vi "IMAQ-MWT DMD XY Calibration (HOST).vi"() -> ()   [LabVIEW 2015]
uses:
  Modules/Common/Controls (HOST)/Image Size.ctl
  Modules/Common/Controls (HOST)/REF.ctl
  Modules/Common/Controls (HOST)/Image Queue Bundle.ctl
  Modules/Common/Controls (HOST)/Data to Disk Bundle.ctl
  Modules/Common/Controls (HOST)/FPGA REF (MWT).ctl
  Modules/Common/Controls (HOST)/Experiment Mode.ctl
  Modules/Common/Controls (HOST)/Main States.ctl
  Modules/Common/Controls (HOST)/IMAQ Parameters.ctl
  Modules/Common/Controls (HOST)/File REF.ctl
  <vilib>/vision/Avi.llb/IMAQ AVI2 Refnum.ctl
  <vilib>/Utility/error.llb/Error Cluster From Error Code.vi
  <vilib>/rvi/errors/niLvFpgaAdjustHostInterfaceError.vi
  <vilib>/FPGAPlugInAG/Dynamic/niLvFpga_Close_Dynamic.vi
  <vilib>/Utility/file.llb/Write Delimited Spreadsheet (I64).vi
  <vilib>/rvi/interface/nirviReadWriteControl/nirviReadWriteControl.xnode
  <vilib>/rvi/interface/nirviCloseFPGA/nirviCloseFPGA.xnode
  NiFpgaLv.dll
  <vilib>/rvi/interface/Simulation/niFpgaSimulationCallBeginRW.vi
  <vilib>/Utility/config.llb/NI_LVConfig.lvlib
  <vilib>/vision/NI_Vision_Development_Module.lvlib
  <vilib>/Utility/config.llb/Write Key (U32).vi
panel:
  out "DMD (Center)":cluster{"X":i32, "Y":i32}={"X"=400, "Y"=300}
  out "Cam (Center)":cluster{"X":i32, "Y":i32}
  in  "DMD ( Top/Left)":cluster{"X":i32, "Y":i32}={"X"=295, "Y"=95}
  in  "DMD #":enum16{"DMD1", "DMD2"}(ring)
  in  "Tab Control":enum32{"Setup", "X Axis", "Y Axis"}(tab)
  in  "Image Size":T1={"Height"=3072, "Width"=3200}
  in  "Experiment Mode":T2
  in  "Pixel Intensity Range":cluster{"Low":u8, "High":u8}={"Low"=25, "High"=135}
  in  "Exp. Time (S)":dbl=120.0
  in  "Stop Button":bool
  in  "Go":bool
  in  "Subtract BG":bool=TRUE
  in  "Replay Interval (ms)":u32=1000
  in  "Swap Bytes":bool
  in  "BOX Height":i32=10
  in  "BOX Width":i32=10
  in  "DMD Height":i32=768
  in  "DMD Width":i32=1024
  out "Particle Reports (Pixels)":T3(array[cluster]) {"Orientation" format="%.2f"; "Dimensions"."Height" format="%.2f"; "Dimensions"."Width" format="%.2f"; "Center of Mass"."Y" format="%.2f"; "Center of Mass"."X" format="%.2f"; "Bounding Rect"."Bottom" format="%.2f"; "Bounding Rect"."Right" format="%.2f"; "Bounding Rect"."Top" format="%.2f"; "Bounding Rect"."Left" format="%.2f"; "Number of Holes" format="%.2f"; "Area" format="%.2f"}
  in  "Range":cluster{"Low":sgl, "High":sgl}={"Low"=150.0, "High"=255.0}
  in  "Selection Values":T5(array[cluster])=[{"Measurement Parameter"=18, "Range Lower Value"=50.0, "Range Upper Value"=1000.0, "Range"=FALSE, "Measurement Type"=FALSE}] {"Measurement Parameter" items=["Center of Mass X", "Center of Mass Y", "First Pixel X", "First Pixel Y", "Bounding Rect Left", "Bounding Rect Top", "Bounding Rect Right", "Bounding Rect Bottom", "Max Feret Diameter Start X", "Max Feret Diameter Start Y", "Max Feret Diameter End X", "Max Feret Diameter End Y", "Max Horiz. Segment Length Left", "Max Horiz. Segment Length Right", "Max Horiz. Segment Length Row", "-", "Bounding Rect Width", "Bounding Rect Height", "Bounding Rect Diagonal", "Perimeter", "Convex Hull Perimeter", "Holes' Perimeter", "Max Feret Diameter", "Equivalent Ellipse Major Axis", "Equivalent Ellipse Minor Axis", "Equivalent Ellipse Minor Axis (Feret)", "Equivalent Rect Long Side", "Equivalent Rect Short Side", "Equivalent Rect Diagonal", "Equivalent Rect Short Side (Feret)", "Average Horiz. Segment Length", "Average Vert. Segment Length", "Hydraulic Radius", "Waddel Disk Diameter", "-", "Area", "Holes' Area", "Particle & Holes' Area", "Convex Hull Area", "Image Area", "-", "Number of Holes", "Number of Horiz. Segments", "Number of Vert. Segments", "-", "Orientation", "Max Feret Diameter Orientation", "-", "% Area/Image Area", "% Area/(Particle & Holes' Area)", "Ratio of Equivalent Ellipse Axes", "Ratio of Equivalent Rect Sides", "-", "Elongation Factor", "Compactness Factor", "Heywood Circularity Factor", "Type Factor", "-", "Sum X", "Sum Y", "Sum XX", "Sum XY", "Sum YY", "Sum XXX", "Sum XXY", "Sum XYY", "Sum YYY", "-", "Moment of Inertia XX", "Moment of Inertia XY", "Moment of Inertia YY", "Moment of Inertia XXX", "Moment of Inertia XXY", "Moment of Inertia XYY", "Moment of Inertia YYY", "Norm. Moment of Inertia XX", "Norm. Moment of Inertia XY", "Norm. Moment of Inertia YY", "Norm. Moment of Inertia XXX", "Norm. Moment of Inertia XXY", "Norm. Moment of Inertia XYY", "Norm. Moment of Inertia YYY", "Hu Moment 1", "Hu Moment 2", "Hu Moment 3", "Hu Moment 4", "Hu Moment 5", "Hu Moment 6", "Hu Moment 7"]; "Range Lower Value" format="%.2f"; "Range Upper Value" format="%.2f"}
  out "Number of Particles":i32
  out "Frame #":u32
  out "Frame Rate":u32
  in  "Movie File Path":path=path "E:/Rawdata/72F11-Gal4xUAS-CsChrimson_20180513_192634.dbde"
  in  "DMD (X Axis)":i32[][](array[numeric])=[[300, 100], [900, 100], [900, 650], [300, 650]]
  in  "Camera (X Axis)":i32[][](array[numeric])
  in  "Save X Table":bool
  in  "Save GUI Parameters":bool
  in  "Gamma":dbl=0.2 format="%#_13g"
  in  "Min Contour Points":u16=127
  in  "N Spine Points":fxp<+,8,8>=41.0
  in  "BG SUB TH":i16=10
  in  "Save Y Table":bool
  in  "DMD (Y Axis)":i32[][](array[numeric])=[[500, 100], [500, 200], [500, 300], [500, 400], [500, 500], [500, 600], [500, 700], [500, 800]]
  in  "Camera (Y Axis)":i32[][](array[numeric])
  out "Exp. Status":string="Camera Connected"
  out "REF":T6
  out "Command Q":refnum<queue>
  out "Display":T9(plugin-control)
  out "Stopped?":bool
  # "DMD XY Calibration"
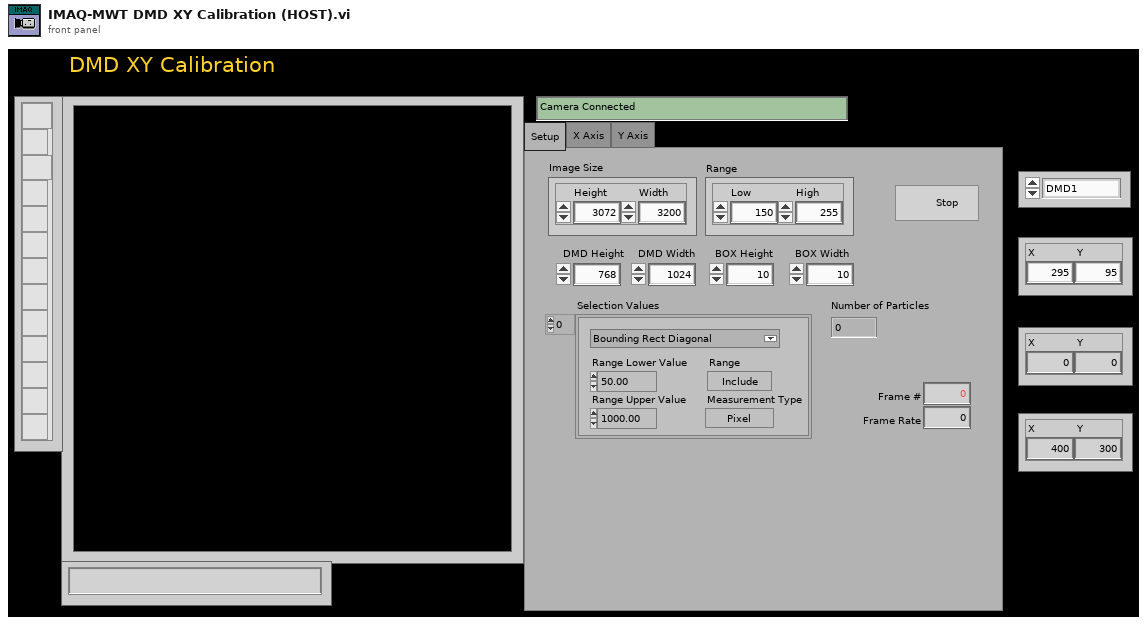
[diagram p1: front panel]
types:
  T1 = typedef "Image Size.ctl" = cluster{"Height":u16, "Width":u16}
  T2 = typedef "Experiment Mode.ctl" = enum16{"Live", "Replay"}
  T3 = cluster{"Area":dbl, "Number of Holes":dbl, "Bounding Rect":cluster{"Left":dbl, "Top":dbl, "Right":dbl, "Bottom":dbl}, "Center of Mass":cluster{"X":dbl, "Y":dbl}, "Orientation":dbl, "Dimensions":cluster{"Width":dbl, "Height":dbl}}[]
  T4 = typedef "Particle Parameters" = i32
  T5 = cluster{"Measurement Parameter":T4, "Range Lower Value":dbl, "Range Upper Value":dbl, "Range":bool, "Measurement Type":bool}[]
  T6 = typedef "REF.ctl" = cluster{"Queue REF":T7, "FPGA REF (MWT)":T8}
  T7 = typedef "Image Queue Bundle.ctl" = cluster{"Disk Image":refnum<queue>, "Image Blocks":refnum<queue>, "Display Image":refnum<queue>, "BG Image":refnum<queue>, "Tag Image":refnum<queue>}
  T8 = typedef "FPGA REF (MWT).ctl" = refnum<k20>
  T9 = typedef "IMAQ Image.ctl" = refnum<image>
  T10 = enum8{"Enabled", "Disabled", "Disabled and Grayed Out"}
  T11 = typedef "Main States.ctl" = enum16{"Open FPGA", "Initialize", "Preview", "Acquire Images", "STOP"}
  T12 = typedef "IMAQ Parameters.ctl" = cluster{"File REF":T13, "Frame Data":cluster{"Width":u32, "Height":u32, "Frames Per Second":u32, "Codec":string}, "File Type":string, "Experiment Mode":T2, "Movie File Path":path}
  T13 = typedef "File REF.ctl" = cluster{"AVI REF":T14, "DBDE REF":refnum<file>}
  T14 = typedef "IMAQ AVI2 Refnum.ctl" = refnum<k20>
  T15 = typedef "Data to Disk Bundle.ctl" = cluster{"Frame Number":u64, "Time Stamp (us)":u64, "Image Data":u64[], "Contour":u32[], "Raw Image REF":refnum<data-value>, "Block Image REF":refnum<data-value>, "Block Box":u64[], "SPINE":u32[], "HT Angle":u64[], "Block Position":u64[], "SPINE Count":u32[], "Contour Count":u32[], "SPINE DIR":u8[]}
  T16 = cluster{"Area":dbl, "Number of Holes":dbl, "Bounding Rect":cluster{"Left":dbl, "Top":dbl, "Right":dbl, "Bottom":dbl}, "Center of Mass":cluster{"X":dbl, "Y":dbl}, "Orientation":dbl, "Dimensions":cluster{"Width":dbl, "Height":dbl}}
  T17 = cluster{"Left":dbl, "Top":dbl, "Right":dbl, "Bottom":dbl}
  T18 = typedef "NI_LVConfig.lvlib/Config Data RefNum.ctl" = refnum<k1>
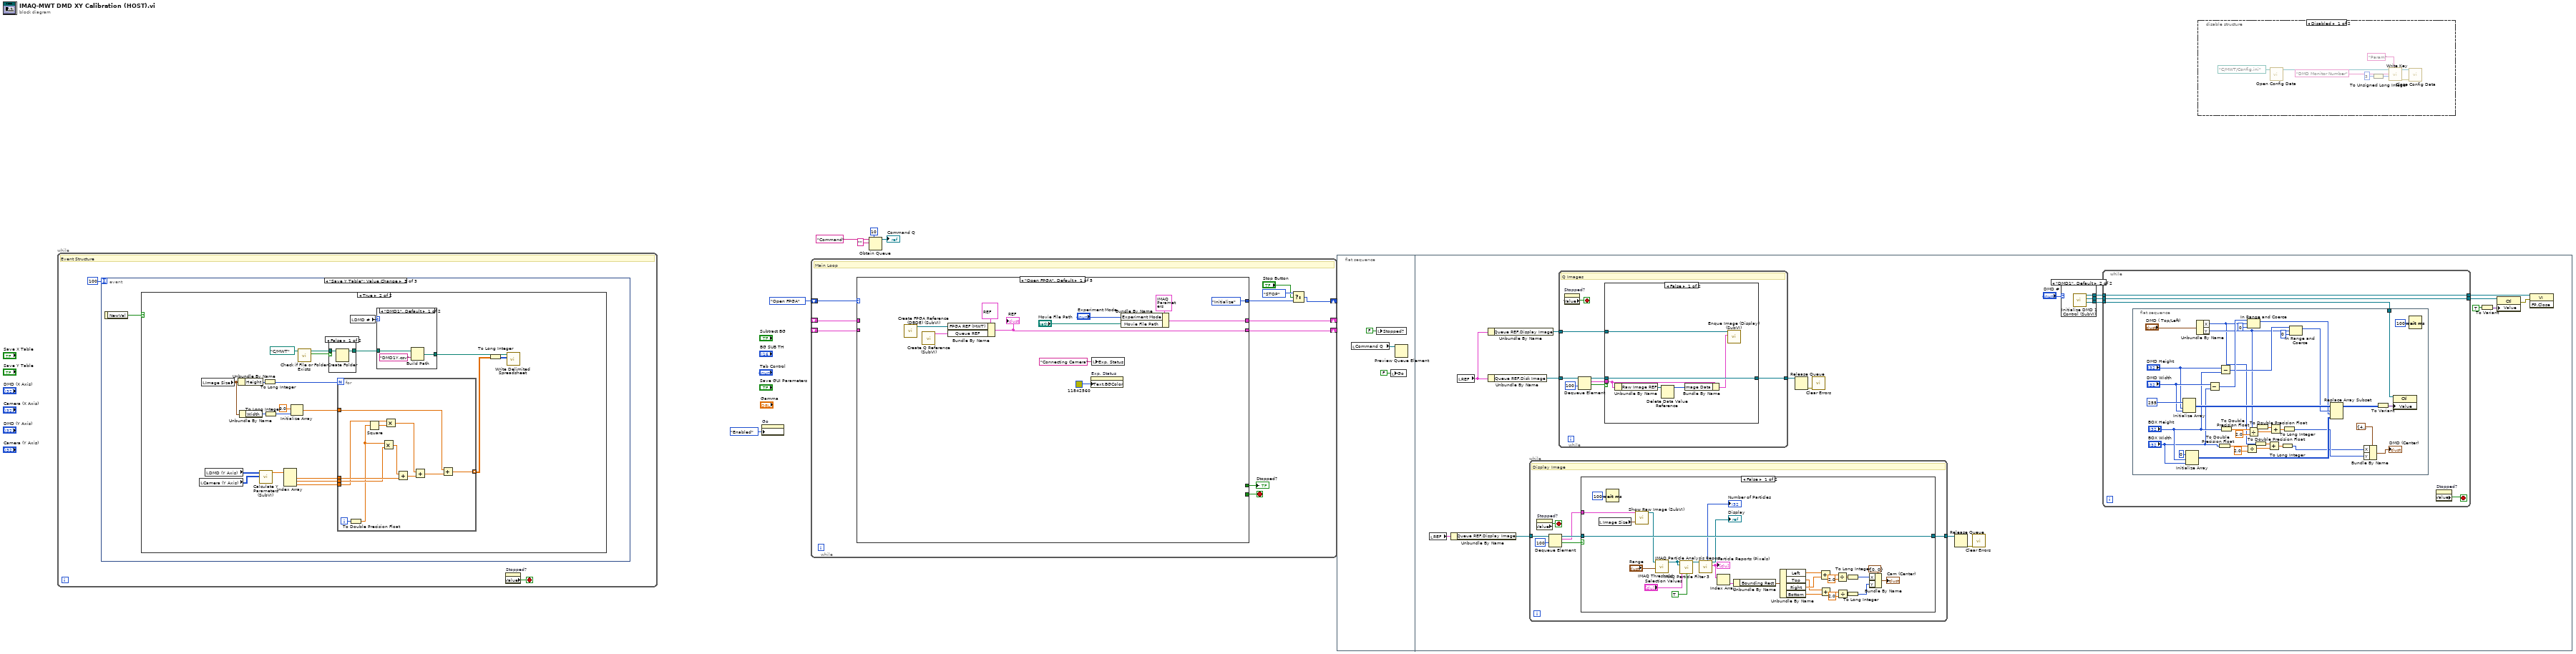
[diagram p0: block diagram]
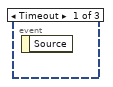
[diagram p2: hidden frame]
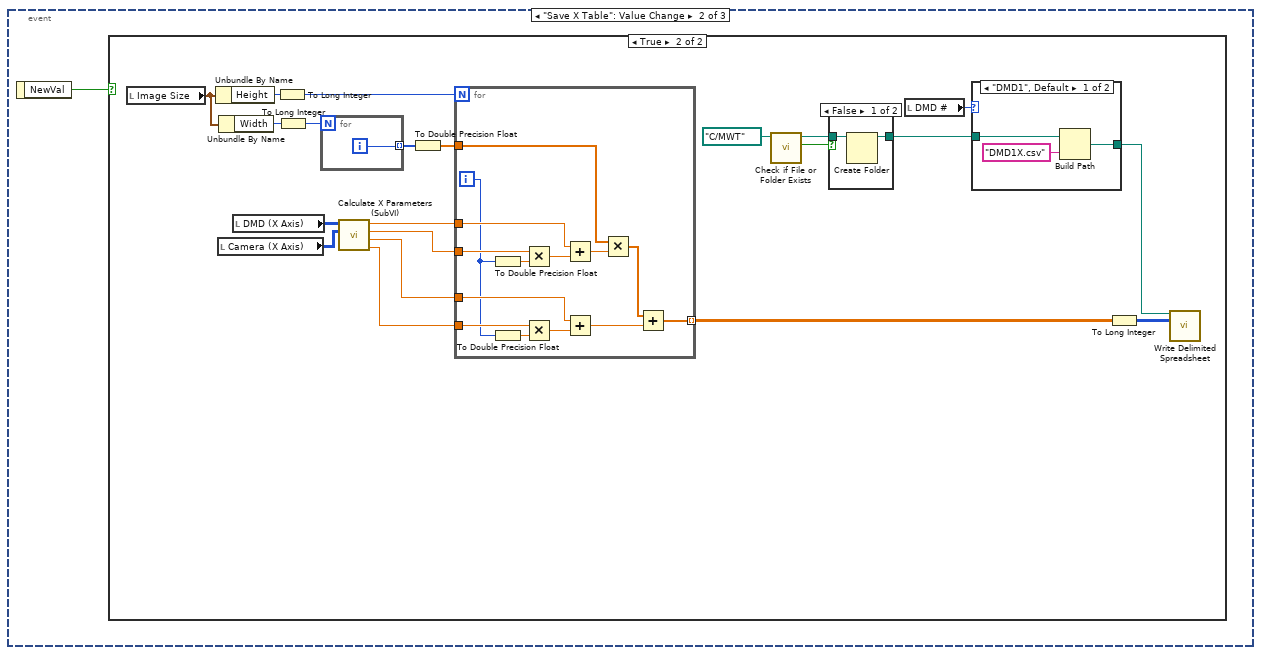
[diagram p3: hidden frame]
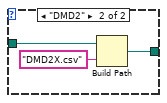
[diagram p6: hidden frame]
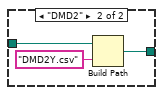
[diagram p9: hidden frame]
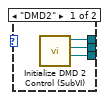
[diagram p11: hidden frame]
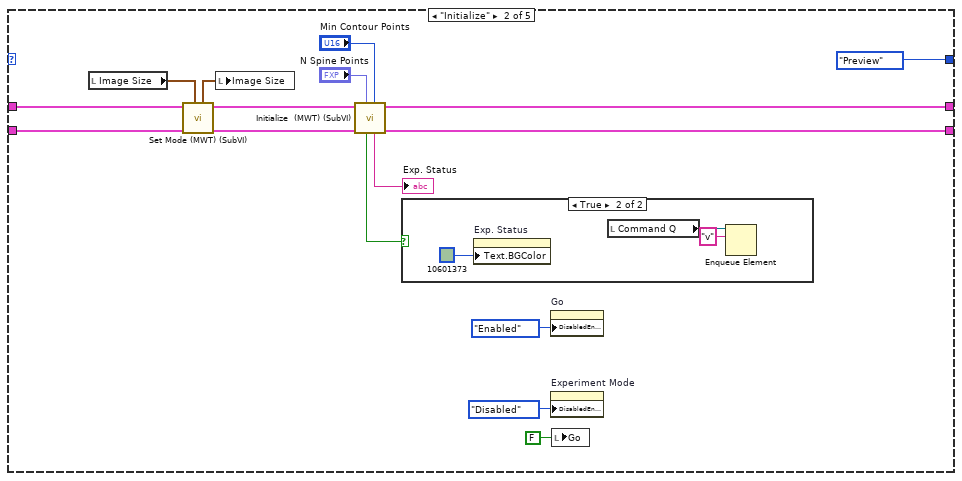
[diagram p14: hidden frame]
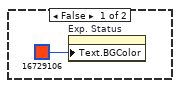
[diagram p15: hidden frame]
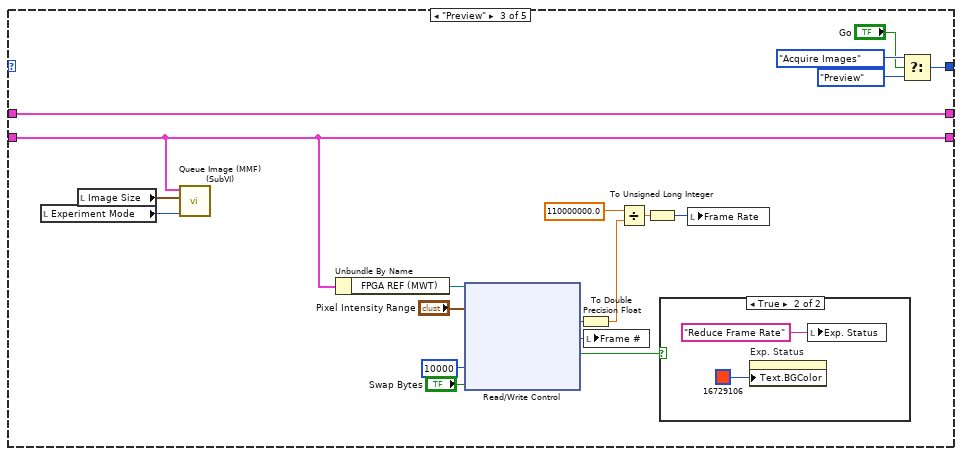
[diagram p16: hidden frame]
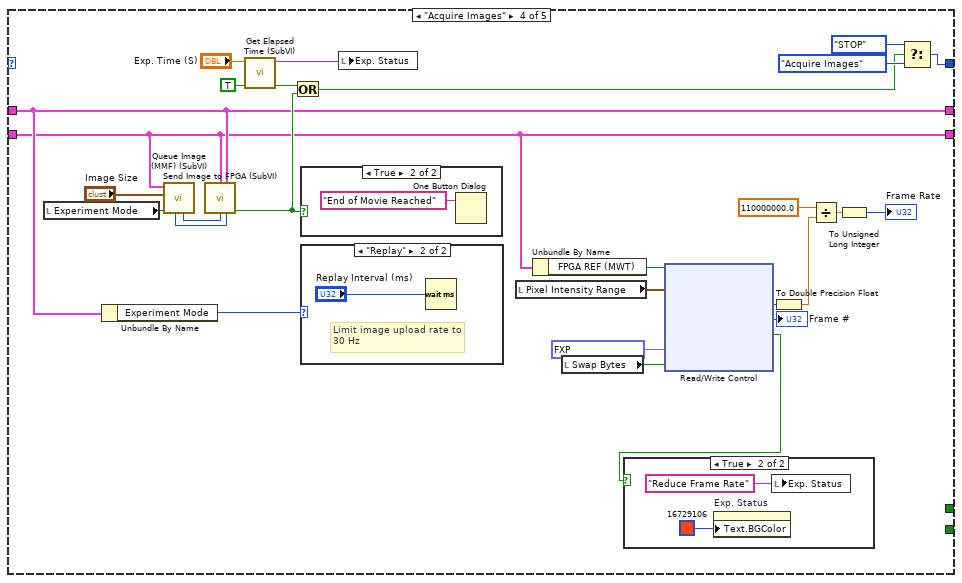
[diagram p18: hidden frame]
diagram:
  n1 = while {
    stop <- w8 stop-if-true
    # "Event Structure"
    n2 = event shown="[2] \"Save Y Table\": Value Change" {
      selector: _ -> [_ _ _]
      dyn-events: _ -> [_ _ _]
      timeout: 100 -> [_ _ _]
      event Timeout {
        n3 = event-data() -> ()  [unwired: 1 in, 1 out]
      }
      event "Save X Table": Value Change {
        n4 = event-data() -> ("NewVal"=w9:bool)  [unwired: 1 in]
        n5 = case shown="True" w9 {
          frame False {
          }
          frame True {
            n6 = local read "Image Size"() -> (w18:T1)
            n7 = Unbundle By Name(w18) -> ("Height"=w30:u16)
            n8 = local read "Camera (X Axis)"() -> (w24:i32[][])
            n9 = Unbundle By Name(w18) -> ("Width"=w28:u16)
            n10 = local read "DMD (X Axis)"() -> (w23:i32[][])
            n11 = To Long Integer(number=w30) -> (32bit integer=w29:i32)
            n12 = To Long Integer(number=w28) -> (32bit integer=w27:i32)
            n13 = for {
              N: w27 -> [_]
              tunnel: [w40] -> w26 mode=indexing
              i -> [w40]
            }
            n14 = call "Calculate X Parameters (SubVI).vi"("Camera"=w24, "DMD"=w23) -> ("Intercept Rate"=w19:dbl, "Intercept"=w20:dbl, "Slope Rate"=w21:dbl, "Slope"=w22:dbl)  [unwired: 6 in]
            n15 = To Double Precision Float(number=w26) -> (double precision float=w25:dbl[])
            n16 = for {
              N: w29 -> [_]
              tunnel: w25 -> [w49]
              tunnel: w22 -> [w51]
              tunnel: w21 -> [w54]
              tunnel: w20 -> [w48]
              tunnel: w19 -> [w45]
              tunnel: [w41] -> w17 mode=indexing
              i -> [w44]
              n17 = To Double Precision Float(number=w44) -> (double precision float=w53:dbl)
              n18 = To Double Precision Float(number=w44) -> (double precision float=w46:dbl)
              n19 = Multiply(x=w54, y=w53) -> (x*y=w52:dbl)
              n20 = Multiply(x=w45, y=w46) -> (x*y=w47:dbl)
              n21 = Add(x=w51, y=w52) -> (x+y=w50:dbl)
              n22 = Add(x=w48, y=w47) -> (x+y=w43:dbl)
              n23 = Multiply(x=w49, y=w50) -> (x*y=w42:dbl[])
              n24 = Add(x=w42, y=w43) -> (x+y=w41:dbl[])
            }
            n25 = call <vilib>:"Check if File or Folder Exists.vi"("path"=path "C:/MWT") -> ("file or folder exists?"=w14:bool, "dup path"=w13:path)  [unwired: 8 in, 1 out]
            n26 = case shown="False" w14 {
              tunnel: w13 -> [w32 w33]
              tunnel: [w31 w33] -> w12
              frame False {
                n27 = Create Folder(path (use dialog)=w32) -> (created path=w31:path)  [unwired: 2 in, 2 out]
              }
              frame True {
              }
            }
            n28 = local read "DMD #"() -> (w16:enum16{"DMD1", "DMD2"})
            n29 = case shown="\"DMD1\", Default" w16 {
              tunnel: w12 -> [w36 w39]
              tunnel: [w34 w37] -> w11
              frame "DMD1", Default {
                n30 = Build Path(base path=w36, name or relative path="DMD1X.csv") -> (appended path=w34:path)
              }
              frame "DMD2" {
                n31 = Build Path(base path=w39, name or relative path="DMD2X.csv") -> (appended path=w37:path)
              }
            }
            n32 = To Long Integer(number=w17) -> (32bit integer=w10:i32[][])
            n33 = call-poly <vilib>:"Write Delimited Spreadsheet.vi"("file path (dialog if empty)"=w11, "2D data"=w10) -> ()  [unwired: 12 in, 2 out]
          }
        }
      }
      event "Save Y Table": Value Change {
        n34 = event-data() -> ("NewVal"=w55:bool)  [unwired: 1 in]
        n35 = case shown="True" w55 {
          frame False {
          }
          frame True {
            n36 = local read "Camera (Y Axis)"() -> (w74:i32[][])
            n37 = local read "Image Size"() -> (w70:T1)
            n38 = local read "DMD (Y Axis)"() -> (w75:i32[][])
            n39 = Unbundle By Name(w70) -> ("Height"=w71:u16)
            n40 = Unbundle By Name(w70) -> ("Width"=w73:u16)
            n41 = call "Calculate Y Parameters (SubVI).vi"("Camera"=w74, "DMD"=w75) -> ("Polynomial Coefficients"=w76:dbl[])  [unwired: 9 in]
            n42 = To Long Integer(number=w71) -> (32bit integer=w72:i32)
            n43 = To Long Integer(number=w73) -> (32bit integer=w59:i32)
            n44 = Index Array(array=w76) -> (element #1=w61:dbl, element #2=w60:dbl, element #3=w56:dbl)  [unwired: 3 in]
            n45 = Initialize Array(0.0 ("element"), w59) -> (w57:dbl[])
            n46 = call <vilib>:"Check if File or Folder Exists.vi"("path"=path "C:/MWT") -> ("file or folder exists?"=w66:bool, "dup path"=w65:path)  [unwired: 8 in, 1 out]
            n47 = case shown="False" w66 {
              tunnel: w65 -> [w78 w79]
              tunnel: [w77 w79] -> w64
              frame False {
                n48 = Create Folder(path (use dialog)=w78) -> (created path=w77:path)  [unwired: 2 in, 2 out]
              }
              frame True {
              }
            }
            n49 = for {
              N: w72 -> [_]
              tunnel: [w87] -> w69 mode=indexing
              tunnel: w61 -> [w95]
              tunnel: w60 -> [w94]
              tunnel: w57 -> [w86]
              tunnel: w56 -> [w90]
              i -> [w93]
              n50 = To Double Precision Float(number=w93) -> (double precision float=w92:dbl)
              n51 = Square(x=w92) -> (x^2=w91:dbl)
              n52 = Multiply(x=w92, y=w94) -> (x*y=w97:dbl)
              n53 = Multiply(x=w90, y=w91) -> (x*y=w88:dbl)
              n54 = Add(x=w97, y=w95) -> (x+y=w96:dbl)
              n55 = Add(x=w88, y=w96) -> (x+y=w89:dbl)
              n56 = Add(x=w86, y=w89) -> (x+y=w87:dbl[])
            }
            n57 = local read "DMD #"() -> (w68:enum16{"DMD1", "DMD2"})
            n58 = case shown="\"DMD1\", Default" w68 {
              tunnel: w64 -> [w80 w83]
              tunnel: [w82 w85] -> w63
              frame "DMD1", Default {
                n59 = Build Path(base path=w80, name or relative path="DMD1Y.csv") -> (appended path=w82:path)
              }
              frame "DMD2" {
                n60 = Build Path(base path=w83, name or relative path="DMD2Y.csv") -> (appended path=w85:path)
              }
            }
            n61 = To Long Integer(number=w69) -> (32bit integer=w62:i32[][])
            n62 = call-poly <vilib>:"Write Delimited Spreadsheet.vi"("file path (dialog if empty)"=w63, "2D data"=w62) -> ()  [unwired: 12 in, 2 out]
          }
        }
      }
    }
    n63 = property on="Stopped?" class="Bool (strict)"() -> ("Value"=w8:bool)  [unwired: 2 in, 2 out]
  }
  n64 = property on="Go" class="Bool (strict)"("DisabledEnum"=T10."Enabled" ("Disabled")) -> ()  [unwired: 2 in, 2 out]
  n65 = while {
    shift-right: [w107] -> _
    shift-left: _ -> [w106]
    shift-right: [w98] -> _
    shift-left: Main_States."Open FPGA" -> [w108]
    shift-right: [w100] -> _
    shift-left: _ -> [w99]
    stop <- w104 stop-if-true
    # "Main Loop"
    n66 = case shown="\"Open FPGA\", Default" w108 {
      tunnel: [w116 w122 w143 w166 w196] -> w107
      tunnel: w106 -> [_ w123 w143 w166 w196]
      tunnel: [Main_States."Initialize" Main_States."Preview" w157 w185 Main_States."STOP"] -> w105
      tunnel: [_ _ _ _ w198] -> w104
      tunnel: [_ _ _ _ w198] -> w103
      tunnel: [w110 w127 w150 w169 w195] -> w100
      tunnel: w99 -> [_ w134 w150 w169 w195]
      frame "Open FPGA", Default {
        n67 = call "Create FPGA Reference (DBDE) (SubVI).vi"() -> ("FPGA REF (MWT)"=w118:T8)  [unwired: 11 in]
        n68 = call "Create Q Reference (SubVI).vi"() -> ("Image Queue"=w117:T7)  [unwired: 11 in]
        n69 = Bundle By Name(cluster=T6 {"Queue REF"={"Disk Image"=refnum, "Image Blocks"=refnum, "Display Image"=refnum, "BG Image"=refnum, "Tag Image"=refnum}, "FPGA REF (MWT)"=refnum}, "FPGA REF (MWT)"=w118, "Queue REF"=w117) -> (w116:T6)
        "REF" <- w116
        n70 = property on="Exp. Status" class="Str"("Text.BGColor"=u32 11842560) -> ()  [unwired: 2 in, 2 out]
        n71 = local write "Exp. Status"("Connecting Camera" ("Exp. Status")) -> ()
        n72 = Bundle By Name(cluster=T12 {"File REF"={"AVI REF"=refnum, "DBDE REF"=refnum}, "Frame Data"={"Width"=0, "Height"=0, "Frames Per Second"=0, "Codec"=""}, "File Type"="", "Experiment Mode"=enum."Live", "Movie File Path"=path "D:/Movies Formatted on November 5th 2015/Clip (2) Formatted.raw"} ("Movie File Property"), "Experiment Mode"="Experiment Mode", "Movie File Path"="Movie File Path") -> (w110:T12)
      }
      frame "Initialize" {
        n73 = local read "Image Size"() -> (w125:T1)
        n74 = call "Set Mode (MWT) (SubVI).vi"("Image Size In"=w125, "REF IN"=w123, "Parameters In"=w134) -> ("REF OUT"=w126:T6, "Parameters Out"=w128:T12, "Image Size Out"=w124:T1)  [unwired: 6 in]
        n75 = local write "Image Size"(w124) -> ()
        n76 = call "Initialize  (MWT) (SubVI).vi"("Min Contour Points"="Min Contour Points", "N Spline Points"="N Spine Points", "REF IN"=w126, "Parameters In"=w128) -> ("REF OUT"=w122:T6, "Parameters Out"=w127:T12, "Exp. Status"=→"Exp. Status":string, "OK?"=w130:bool)  [unwired: 4 in]
        n77 = case shown="True" w130 {
          frame False {
            n78 = property on="Exp. Status" class="Str"("Text.BGColor"=u32 16729106) -> ()  [unwired: 2 in, 2 out]
          }
          frame True {
            n79 = property on="Exp. Status" class="Str"("Text.BGColor"=u32 10601373) -> ()  [unwired: 2 in, 2 out]
            n80 = local read "Command Q"() -> (w138:refnum<queue>)
            n81 = Enqueue Element(queue=w138, element="v") -> ()  [unwired: 2 in, 3 out]
          }
        }
        n82 = property on="Go" class="Bool (strict)"("DisabledEnum"=T10."Enabled" ("Disabled")) -> ()  [unwired: 2 in, 2 out]
        n83 = property on="Experiment Mode" class="Enum (strict)"("DisabledEnum"=T10."Disabled" ("Disabled")) -> ()  [unwired: 2 in, 2 out]
        n84 = local write "Go"(FALSE ("Go")) -> ()
      }
      frame "Preview" {
        n85 = local read "Experiment Mode"() -> (w141:T2)
        n86 = local read "Image Size"() -> (w147:T1)
        n87 = call "Queue Image (MMF) (SubVI).vi"("Experiment Mode"=w141, "Image Size"=w147, "Data Bundle"=w143) -> ()  [unwired: 9 in]
        n88 = Unbundle By Name(w143) -> ("FPGA REF (MWT)"=w153:T8)
        n89 = xnode "Read/Write Control"("FPGA VI Reference In"=w153, "Pixel Intensity"="Pixel Intensity Range", "Clock Cycles Limit"=u32 10000, "Swap Bytes"="Swap Bytes") -> ("Frame Interval"=w155:u32, "Frame #"=w146:u32, "DMA Timeout"=w145:bool)  [unwired: 1 in, 2 out]
        n90 = To Double Precision Float(number=w155) -> (double precision float=w154:dbl)
        n91 = local write "Frame #"(w146) -> ()
        n92 = Divide(x=110000000.0 ("y"), y=w154) -> (x/y=w151:dbl)
        n93 = To Unsigned Long Integer(number=w151) -> (unsigned 32bit integer=w149:u32)
        n94 = case shown="True" w145 {
          frame False {
          }
          frame True {
            n95 = property on="Exp. Status" class="Str"("Text.BGColor"=u32 16729106) -> ()  [unwired: 2 in, 2 out]
            n96 = local write "Exp. Status"("Reduce Frame Rate" ("Exp. Status")) -> ()
          }
        }
        n97 = local write "Frame Rate"(w149) -> ()
        n98 = Select(t=Main_States."Acquire Images", s="Go", f=Main_States."Preview") -> (s? t:f=w157:T11)
      }
      frame "Acquire Images" {
        n99 = local read "Experiment Mode"() -> (w164:T2)
        n100 = Unbundle By Name(w169) -> ("Experiment Mode"=w168:T2)
        n101 = call "Send Image to FPGA (SubVI).vi"("Data Bundle"=w166, "Parameters"=w169) -> ("TimeStamp"=w163:u64, "Frame Number"=w162:u64, "EOF"=w183:bool)  [unwired: 11 in]
        n102 = call "Queue Image (MMF) (SubVI).vi"("TimeStamp"=w163, "Frame Number"=w162, "Experiment Mode"=w164, "Image Size"="Image Size", "Data Bundle"=w166) -> ()  [unwired: 7 in]
        n103 = call "Get Elapsed Time (SubVI).vi"("Go"=TRUE, "Experiment Time (S)"="Exp. Time (S)") -> ("Done"=w174:bool, "Time Status"=w173:string)  [unwired: 8 in]
        n104 = Or(x=w174, y=w183) -> (x .or. y?=w175:bool)
        n105 = case shown="True" w183 {
          frame False {
          }
          frame True {
            n106 = One Button Dialog(message="End of Movie Reached") -> ()  [unwired: 1 in, 1 out]
          }
        }
        n107 = case shown="\"Replay\"" w168 {
          frame "Live", Default {
          }
          frame "Replay" {
            # "Limit image upload rate to 30 Hz"
            n108 = Wait (ms)(milliseconds to wait="Replay Interval (ms)") -> ()  [unwired: 1 out]
          }
        }
        n109 = local write "Exp. Status"(w173) -> ()
        n110 = local read "Pixel Intensity Range"() -> (w167:cluster{"Low":u8, "High":u8})
        n111 = Unbundle By Name(w166) -> ("FPGA REF (MWT)"=w180:T8)
        n112 = local read "Swap Bytes"() -> (w161:bool)
        n113 = xnode "Read/Write Control"("FPGA VI Reference In"=w180, "Pixel Intensity"=w167, "Significant Angle"=fxp<+,16,3> 0.0699462890625, "Swap Bytes"=w161) -> ("Frame Interval"=w182:u32, "Frame #"=→"Frame #":u32, "DMA Timeout"=w170:bool)  [unwired: 1 in, 2 out]
        n114 = case shown="True" w170 {
          frame False {
          }
          frame True {
            n115 = property on="Exp. Status" class="Str"("Text.BGColor"=u32 16729106) -> ()  [unwired: 2 in, 2 out]
            n116 = local write "Exp. Status"("Reduce Frame Rate" ("Exp. Status")) -> ()
          }
        }
        n117 = To Double Precision Float(number=w182) -> (double precision float=w181:dbl)
        n118 = Divide(x=110000000.0 ("y"), y=w181) -> (x/y=w177:dbl)
        n119 = To Unsigned Long Integer(number=w177) -> (unsigned 32bit integer=→"Frame Rate":u32)
        n120 = Select(t=Main_States."STOP", s=w175, f=Main_States."Acquire Images") -> (s? t:f=w185:T11)
      }
      frame "STOP" {
        w198 = TRUE
        n121 = Unbundle By Name(w196) -> ("FPGA REF (MWT)"=w197:T8)
        n122 = xnode "Close FPGA VI Reference"("FPGA VI Reference In"=w197) -> ("error out"=w192:errorcluster)  [unwired: 1 in]
        n123 = call <vilib>:"Clear Errors.vi"("error in (no error)"=w192) -> ()  [unwired: 5 in, 2 out]
        n124 = local write "Exp. Status"("Experiment Complete!" ("Exp. Status")) -> ()
        n125 = property on="Experiment Mode" class="Enum (strict)"("DisabledEnum"=T10."Enabled" ("Disabled")) -> ()  [unwired: 2 in, 2 out]
      }
    }
    "Stopped?" <- w103
    n126 = Select(t=Main_States."STOP", s="Stop Button", f=w105) -> (s? t:f=w98:T11)
  }
  n127 = Obtain Queue(max queue size (-1, unlimited)=10, name (unnamed)="Command", element data type="" ("name (unnamed)")) -> (queue out=→"Command Q":refnum<queue>)  [unwired: 2 in, 2 out]
  n128 = flat-sequence {
    frame #0 {
      n129 = local read "Command Q"() -> (w202:refnum<queue>)
      n130 = local write "Stopped?"(FALSE ("Stopped?")) -> ()
      n131 = local write "Go"(FALSE ("Go")) -> ()
      n132 = Preview Queue Element(queue=w202) -> ()  [unwired: 2 in, 4 out]
    }
    frame #1 {
      n133 = local read "REF"() -> (w219:T6)
      n134 = Unbundle By Name(w219) -> ("Queue REF.Display Image"=w218:refnum<queue>)
      n135 = local read "REF"() -> (w214:T6)
      n136 = Unbundle By Name(w214) -> ("Queue REF.Display Image"=w215:refnum<queue>)
      n137 = Unbundle By Name(w214) -> ("Queue REF.Disk Image"=w216:refnum<queue>)
      n138 = while {
        tunnel: [w284] -> w220
        tunnel: w218 -> [w283]
        stop <- w281 stop-if-true
        # "Display Image"
        n139 = property on="Stopped?" class="Bool (strict)"() -> ("Value"=w281:bool)  [unwired: 2 in, 2 out]
        n140 = Dequeue Element(queue=w283, timeout in ms (-1)=100) -> (queue out=w285:refnum<queue>, element=w282:T15, timed out?=w286:bool)  [unwired: 1 in, 1 out]
        n141 = case shown="False" w286 {
          tunnel: w285 -> [w316 w317]
          tunnel: [w316 w317] -> w284
          tunnel: w282 -> [w315 _]
          frame False {
            n142 = local read "Image Size"() -> (w313:T1)
            n143 = Wait (ms)(milliseconds to wait=u32 100) -> ()  [unwired: 1 out]
            n144 = call "Show Raw Image (SubVI).vi"("Display Data"=w315, "Image Size"=w313) -> ("Image Out"=w312:T9)  [unwired: 17 in]
            n145 = call "IMAQ Threshold"("Range"="Range", "Image Src"=w312) -> ("Image Dst Out"=w311:T9)  [unwired: 8 in, 1 out]
            n146 = call "IMAQ Particle Filter 3"("Image Src"=w311, "Image Dst"=w311, "Selection Values"="Selection Values", "Fill Holes? (F)"=TRUE) -> ("Image Dst Out"=w309:T9)  [unwired: 9 in, 2 out]
            n147 = call "IMAQ Particle Analysis Report"("Image"=w309) -> ("Particle Reports (Pixels)"=w307:T3, "Image Out (duplicate)"=→"Display":T9, "Number of Particles"=→"Number of Particles":i32)  [unwired: 5 in, 3 out]
            "Particle Reports (Pixels)" <- w307
            n148 = Index Array(array=w307) -> (element=w306:T16)  [unwired: 1 in]
            n149 = Unbundle By Name(w306) -> ("Bounding Rect"=w305:T17)
            n150 = Unbundle By Name(w305) -> ("Left"=w304:dbl, "Top"=w297:dbl, "Right"=w303:dbl, "Bottom"=w298:dbl)
            n151 = Add(x=w304, y=w303) -> (x+y=w302:dbl)
            n152 = Add(x=w297, y=w298) -> (x+y=w299:dbl)
            n153 = Divide(x=w302, y=2.0) -> (x/y=w296:dbl)
            n154 = Divide(x=w299, y=2.0) -> (x/y=w295:dbl)
            n155 = To Long Integer(number=w296) -> (32bit integer=w291:i32)
            n156 = To Long Integer(number=w295) -> (32bit integer=w290:i32)
            n157 = Bundle By Name(cluster=cluster{"X":i32, "Y":i32} {"X"=0, "Y"=0}, "X"=w291, "Y"=w290) -> (→"Cam (Center)":cluster{"X":i32, "Y":i32})
          }
          frame True {
          }
        }
      }
      n158 = while {
        tunnel: [w272] -> w217
        tunnel: w216 -> [w266]
        tunnel: w215 -> [w271]
        stop <- w267 stop-if-true
        # "Q Images"
        n159 = property on="Stopped?" class="Bool (strict)"() -> ("Value"=w267:bool)  [unwired: 2 in, 2 out]
        n160 = Dequeue Element(queue=w266, timeout in ms (-1)=100) -> (queue out=w269:refnum<queue>, element=w270:T15, timed out?=w268:bool)  [unwired: 1 in, 1 out]
        n161 = case shown="False" w268 {
          tunnel: w269 -> [w279 w280]
          tunnel: [w279 w280] -> w272
          tunnel: w271 -> [w278 _]
          tunnel: w270 -> [w276 _]
          frame False {
            n162 = Unbundle By Name(w276) -> ("Raw Image REF"=w277:refnum<data-value>)
            n163 = Delete Data Value Reference(data value reference=w277) -> (data value=w275:u64[])  [unwired: 1 in, 1 out]
            n164 = Bundle By Name(cluster=w276, "Image Data"=w275) -> (w274:T15)
            n165 = call "Enque Image (Display) (SubVI).vi"("Data Bundle"=w274, "Display Image REF"=w278) -> ()  [unwired: 10 in]
          }
          frame True {
          }
        }
      }
      n166 = Release Queue(queue=w217) -> (error out=w212:errorcluster)  [unwired: 2 in, 2 out]
      n167 = call <vilib>:"Clear Errors.vi"("error in (no error)"=w212) -> ()  [unwired: 5 in, 2 out]
      n168 = Release Queue(queue=w220) -> (error out=w213:errorcluster)  [unwired: 2 in, 2 out]
      n169 = call <vilib>:"Clear Errors.vi"("error in (no error)"=w213) -> ()  [unwired: 5 in, 2 out]
      n170 = case shown="\"DMD1\", Default" "DMD #" {
        tunnel: [w223 w226] -> w211
        tunnel: [w222 w225] -> w210
        tunnel: [w221 w224] -> w204
        frame "DMD2" {
          n171 = call "Initialize DMD 2 Control (SubVI).vi"() -> ("DMD IMG REF"=w221:refnum<vi>, "STOP REF"=w222:refnum<vi>, "DMD VI REF"=w223:refnum<vi>)  [unwired: 9 in]
        }
        frame "DMD1", Default {
          n172 = call "Initialize DMD 1 Control (SubVI).vi"() -> ("DMD IMG REF"=w224:refnum<vi>, "STOP REF"=w225:refnum<vi>, "DMD VI REF"=w226:refnum<vi>)  [unwired: 9 in]
        }
      }
      n173 = while {
        tunnel: w211 -> [w228]
        tunnel: w210 -> [w229]
        tunnel: [w229] -> w208
        tunnel: [w228] -> w205
        tunnel: w204 -> [w227]
        stop <- w230 stop-if-true
        n174 = flat-sequence {
          tunnel: w227 -> [w263]
          frame #0 {
            n175 = Initialize Array(u8 255 ("element"), "DMD Height", "DMD Width") -> (w258:u8[][])
            n176 = Initialize Array(u8 0 ("element"), "BOX Height", "BOX Width") -> (w260:u8[][])
            n177 = Unbundle By Name("DMD ( Top/Left)") -> ("X"=w231:i32, "Y"=w244:i32)
            n178 = Subtract(x="DMD Width", y="BOX Width") -> (x-y=w255:i32)
            n179 = To Double Precision Float(number="BOX Width") -> (double precision float=w235:dbl)
            n180 = Subtract(x="DMD Height", y="BOX Height") -> (x-y=w251:i32)
            n181 = To Double Precision Float(number="BOX Height") -> (double precision float=w246:dbl)
            n182 = Divide(x=w235, y=2.0) -> (x/y=w236:dbl)
            n183 = In Range and Coerce(upper limit=w255, x=w231, lower limit=0) -> (coerced(x)=w249:i32)  [unwired: 1 out]
            n184 = Divide(x=w246, y=2.0) -> (x/y=w245:dbl)
            n185 = To Double Precision Float(number=w231) -> (double precision float=w237:dbl)
            n186 = To Double Precision Float(number=w244) -> (double precision float=w243:dbl)
            n187 = Add(x=w237, y=w236) -> (x+y=w238:dbl)
            n188 = Add(x=w243, y=w245) -> (x+y=w240:dbl)
            n189 = To Long Integer(number=w238) -> (32bit integer=w232:i32)
            n190 = To Long Integer(number=w240) -> (32bit integer=w239:i32)
            n191 = In Range and Coerce(upper limit=w251, x=w244, lower limit=0) -> (coerced(x)=w250:i32)  [unwired: 1 out]
            n192 = Replace Array Subset(array=w258, new element=w260, index (row)=w250, index (col)=w249) -> (w265:u8[][])
            n193 = Bundle By Name(cluster=cluster{"X":i32, "Y":i32} {"X"=400, "Y"=300} ("DMD (Center)"), "X"=w232, "Y"=w239) -> (→"DMD (Center)":cluster{"X":i32, "Y":i32})
            n194 = To Variant(anything=w265) -> (Variant=w264:variant)
            n195 = property class="Ctl"(reference=w263, "Value"=w264) -> ()  [unwired: 1 in, 2 out]
            n196 = Wait (ms)(milliseconds to wait=u32 100) -> ()  [unwired: 1 out]
          }
        }
        n197 = property on="Stopped?" class="Bool (strict)"() -> ("Value"=w230:bool)  [unwired: 2 in, 2 out]
      }
      n198 = To Variant(anything=TRUE ("Wait Until Done")) -> (Variant=w209:variant)
      n199 = property class="Ctl"(reference=w208, "Value"=w209) -> (error out=w206:errorcluster)  [unwired: 1 in, 1 out]
      n200 = invoke class="VI" method="FP.Close"(reference=w205, error in=w206) -> ()  [unwired: 1 in, 3 out]
    }
  }
  n201 = disable-structure shown="Disabled" {
    frame Disabled {
      n202 = call <vilib>:"Open Config Data.vi"("configuration file path"=path "C:/MWT/Config.ini") -> ("refnum"=w322:T18)  [unwired: 8 in, 2 out]
      n203 = To Unsigned Long Integer(number=u16 3 ("Front Panel Window:Monitor")) -> (unsigned 32bit integer=w321:u32)
      n204 = call-poly <vilib>:"Write Key.vi"("section"="Param", "value"=w321, "key"="DMD Monitor Number" ("section"), "refnum"=w322) -> ("error out"=w319:errorcluster, "refnum out"=w318:T18)  [unwired: 5 in, 1 out]
      n205 = call <vilib>:"Close Config Data.vi"("error in (no error)"=w319, "refnum"=w318) -> ()  [unwired: 8 in, 2 out]
    }
    frame Enabled {
    }
  }
